vi "Read Motor Controller IDs 2.vi"(8 "error in (no error)":errorcluster, 11 "Tank Drive in":refnum<class "Tank Drive.lvclass">) -> (0 "error out":errorcluster, 2 "Motor Controller IDs":T1, 3 "Tank Drive out":refnum<class "Tank Drive.lvclass">)   [LabVIEW 2019, in "Drive.lvlib" / "Tank Drive.lvclass"]
uses:
  Tank Drive.lvclass
  Controls/Motor Controller IDs.ctl
  Tank Drive.lvclass/Tank Drive.ctl
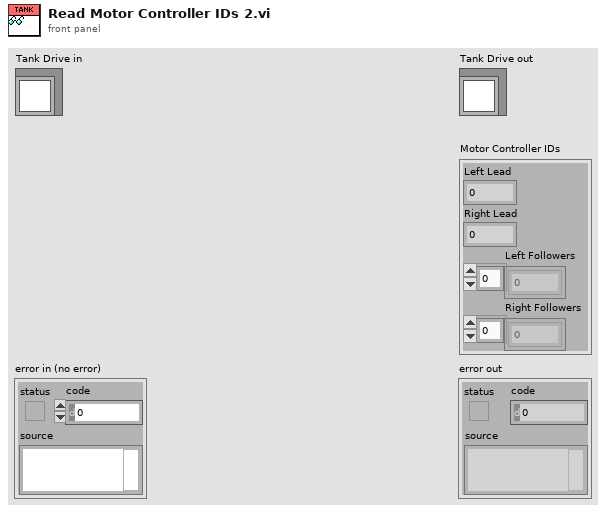
[diagram p1: front panel]
types:
  T1 = typedef "Drive.lvlib/Tank Drive.lvclass/Motor Controller IDs.ctl" = cluster{"Left Lead":u8, "Right Lead":u8, "Left Followers":u8[], "Right Followers":u8[]}
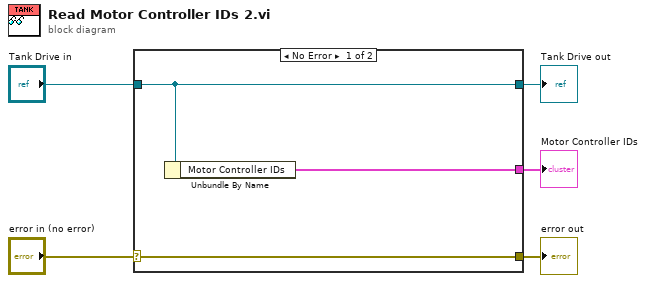
[diagram p0: block diagram]
diagram:
  n1 = case shown="No Error" "error in (no error)" {
    selector: "error in (no error)" -> [w8 w9]
    tunnel: [w8 w9] -> w4
    tunnel: [w7 w10] -> w2
    tunnel: "Tank Drive in" -> [w7 w10]
    tunnel: [w6 _] -> w1
    frame No Error {
      n2 = Unbundle By Name(w7) -> ("Motor Controller IDs"=w6:T1)
    }
    frame Error {
    }
  }
  "error out" <- w4
  "Tank Drive out" <- w2
  "Motor Controller IDs" <- w1
